vi "Hide My Panel.vi"(8 "error in (no error)":errorcluster, 11 "Panel Actor in":refnum<class "Panel Actor.lvclass">) -> (0 "error out":errorcluster, 3 "Panel Actor out":refnum<class "Panel Actor.lvclass">)   [LabVIEW 2017, in "MGI-Panel Actor.lvlib" / "Panel Actor.lvclass"]
doc: "Hides the panel.\n\n----\nCopyright: MGI 2018\nAuthor: Derek Trepanier"
uses:
  Panel Actor.lvclass
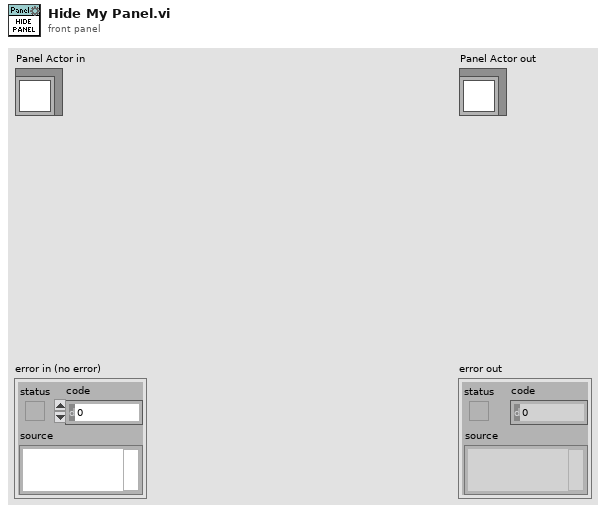
[diagram p1: front panel]
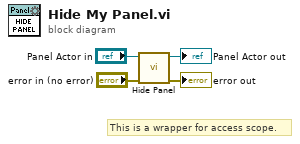
[diagram p0: block diagram]
diagram:
  # "This is a wrapper for access scope."
  n1 = call "Hide Panel.vi"("error in (no error)"="error in (no error)", "Panel Actor in"="Panel Actor in") -> ("error out"=→"error out":errorcluster, "Panel Actor out"=→"Panel Actor out":refnum<class "Panel Actor.lvclass">)  [unwired: 8 in]
